vi "Stim Pulse Generator.vi"() -> ()   [LabVIEW 2020]
uses:
  <vilib>/Waveform/WDTOps.llb/WDT Append Waveforms DBL.vi
  <vilib>/measure/NI_MABase.lvlib
panel:
  out "Waveform Graph":waveform(dbl)(graph)
  in  "Pulse\nAmplitude (mA)":dbl
  in  "Pulse\nFrequency (Hz)":u32
  in  "Pulse\nDuration (µs)":dbl
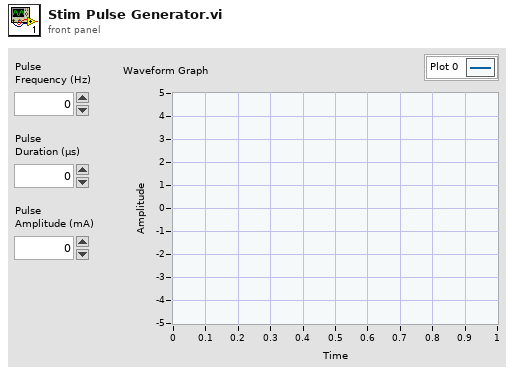
[diagram p1: front panel]
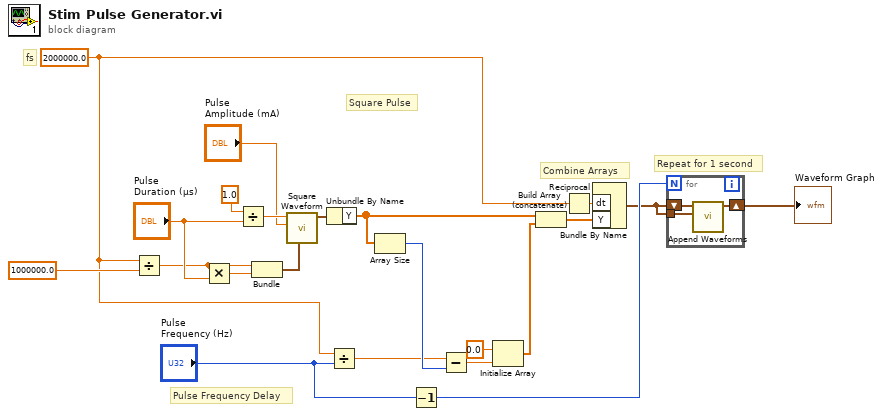
[diagram p0: block diagram]
diagram:
  w1 = 2000000.0 ("x")
  # "fs"
  # "Repeat for 1 second"
  # "Combine Arrays"
  # "Pulse Frequency Delay"
  # "Square Pulse"
  n1 = Divide(x=w1, y=1000000.0) -> (x/y=w3:dbl)
  n2 = Multiply(x=w3, y="Pulse\nDuration (µs)") -> (x*y=w19:dbl)
  n3 = Divide(x=1.0, y="Pulse\nDuration (µs)") -> (x/y=w21:dbl)
  n4 = Bundle(w3, w19) -> (w22:cluster{dbl, dbl})  [unwired: 1 in]
  n5 = call <vilib>:"Square Waveform.vi"("sampling info"=w22, "amplitude"="Pulse\nAmplitude (mA)", "frequency"=w21) -> ("signal out"=w16:waveform(dbl))  [unwired: 7 in, 1 out]
  n6 = Unbundle By Name(w16) -> ("Y"=w11:dbl[])
  n7 = Divide(x=w1, y="Pulse\nFrequency (Hz)") -> (x/y=w13:dbl)
  n8 = Array Size(array=w11) -> (size(s)=w15:i32)
  n9 = Decrement(x="Pulse\nFrequency (Hz)") -> (x-1=w8:u32)
  n10 = Subtract(x=w13, y=w15) -> (x-y=w14:dbl)
  n11 = Initialize Array(0.0 ("element"), w14) -> (w10:dbl[])
  n12 = Build Array (concatenate)(w11, w10) -> (w9:dbl[])
  n13 = Reciprocal(x=w1) -> (1/x=w4:dbl)
  n14 = Bundle By Name("dt"=w4, "Y"=w9) -> (w6:waveform(dbl))  [unwired: 1 in]
  n15 = for {
    N: w8 -> [_]
    tunnel: w6 -> [w24]
    shift-right: [w23] -> w5
    shift-left: w6 -> [w25]
    n16 = call-poly <vilib>:"Append Waveforms.vi"("waveform B"=w24, "waveform A"=w25) -> ("waveform out"=w23:waveform(dbl))  [unwired: 8 in, 1 out]
  }
  "Waveform Graph" <- w5
